vi "list-shared-dependencies.vi"(8 "error in (no error)":errorcluster) -> (0 "error out":errorcluster)   [LabVIEW 2013]
uses:
  src/SMO/SMO.lvclass
  _test-support-SMOs/SMO.SelfTerminatingOverride/SMO.SelfTerminatingOverride.lvclass
  <vilib>/addons/_JKI Toolkits/Caraya/classes/Test/Test.lvclass
  <vilib>/addons/_JKI Toolkits/Caraya/classes/Assert/Assert.lvclass
panel:
  out "[Dependencies] 2":refnum<class "SMO.lvclass">[](array[class])
  out "[Dependencies]":refnum<class "SMO.lvclass">[](array[class])
  # "<< Should have two dependencies"
  # "<< Should have one dependency"
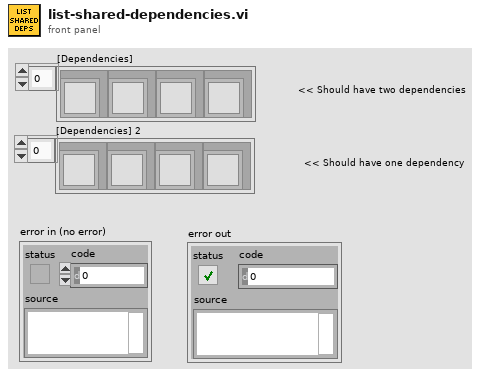
[diagram p1: front panel]
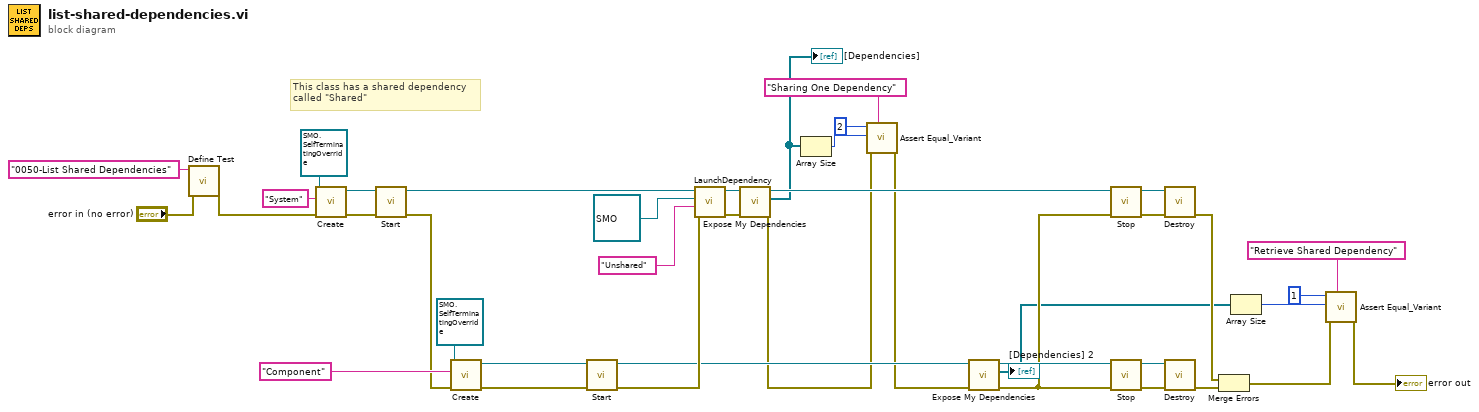
[diagram p0: block diagram]
diagram:
  # "This class has a shared dependency\ncalled \"Shared\""
  n1 = call <vilib>:"Define Test.vi"("error in (no error)"="error in (no error)", "Label (VI Title)"="0050-List Shared Dependencies") -> ("error out"=w13:errorcluster)  [unwired: 9 in]
  n2 = call "Create.vi"("error in (no error)"=w13, "Subsystem Name (optional)"="System", "SMO"=refnum<class "SMO.SelfTerminatingOverride.lvclass"> refnum ("SMO.SelfTerminatingOverride.lvclass")) -> ("error out"=w38:errorcluster, "SMO out"=w39:refnum<class "SMO.SelfTerminatingOverride.lvclass">)  [unwired: 6 in, 1 out]
  n3 = call "Start.vi"("error in (no error)"=w38, "SMO"=w39) -> ("error out"=w31:errorcluster, "SMO out"=w28:refnum<class "SMO.SelfTerminatingOverride.lvclass">)  [unwired: 8 in]
  n4 = call "Create.vi"("error in (no error)"=w31, "Subsystem Name (optional)"="Component", "SMO"=refnum<class "SMO.SelfTerminatingOverride.lvclass"> refnum ("SMO.SelfTerminatingOverride.lvclass")) -> ("error out"=w30:errorcluster, "SMO out"=w32:refnum<class "SMO.SelfTerminatingOverride.lvclass">)  [unwired: 6 in, 1 out]
  n5 = call "Start.vi"("error in (no error)"=w30, "SMO"=w32) -> ("error out"=w24:errorcluster, "SMO out"=w22:refnum<class "SMO.SelfTerminatingOverride.lvclass">)  [unwired: 8 in]
  n6 = call "LaunchDependency.vi"("error in (no error)"=w24, "Dependency Name"="Unshared" ("Subsystem Name (optional)"), "Dependency Type"=refnum<class "SMO.lvclass"> refnum, "SMO in"=w28) -> ("error out"=w23:errorcluster, "SMO out"=w27:refnum<class "SMO.SelfTerminatingOverride.lvclass">)  [unwired: 4 in, 2 out]
  n7 = call "Expose My Dependencies.vi"("error in (no error)"=w23, "SMO.SelfTerminatingOverride in"=w27) -> ("error out"=w2:errorcluster, "[Dependencies]"=w12:refnum<class "SMO.lvclass">[], "SMO.SelfTerminatingOverride out"=w29:refnum<class "SMO.SelfTerminatingOverride.lvclass">)  [unwired: 7 in]
  "[Dependencies]" <- w12
  n8 = Array Size(array=w12) -> (size(s)=w10:i32)
  n9 = call <vilib>:"Assert Equal_Variant.vi"("Label"="Sharing One Dependency" ("Label (VI Title)"), "error in (no error)"=w2, "Y"=w10, "X"=2 ("size(s)")) -> ("error out"=w1:errorcluster)  [unwired: 7 in]
  n10 = call "Expose My Dependencies.vi"("error in (no error)"=w1, "SMO.SelfTerminatingOverride in"=w22) -> ("error out"=w18:errorcluster, "[Dependencies]"=w11:refnum<class "SMO.lvclass">[], "SMO.SelfTerminatingOverride out"=w19:refnum<class "SMO.SelfTerminatingOverride.lvclass">)  [unwired: 7 in]
  "[Dependencies] 2" <- w11
  n11 = call "Stop.vi"("error in (no error)"=w18, "SMO"=w29) -> ("error out"=w35:errorcluster, "SMO out"=w36:refnum<class "SMO.SelfTerminatingOverride.lvclass">)  [unwired: 8 in]
  n12 = call "Stop.vi"("error in (no error)"=w18, "SMO"=w19) -> ("error out"=w21:errorcluster, "SMO out"=w20:refnum<class "SMO.SelfTerminatingOverride.lvclass">)  [unwired: 8 in]
  n13 = call "Destroy.vi"("error in (no error)"=w35, "SMO"=w36) -> ("error out"=w16:errorcluster)  [unwired: 9 in]
  n14 = call "Destroy.vi"("error in (no error)"=w21, "SMO"=w20) -> ("error out"=w17:errorcluster)  [unwired: 9 in]
  n15 = Merge Errors(w16, w17) -> (w6:errorcluster)
  n16 = Array Size(array=w11) -> (size(s)=w7:i32)
  n17 = call <vilib>:"Assert Equal_Variant.vi"("Label"="Retrieve Shared Dependency" ("Label (VI Title)"), "error in (no error)"=w6, "Y"=w7, "X"=1 ("size(s)")) -> ("error out"=→"error out":errorcluster)  [unwired: 7 in]
